vi "Problemas de Monitoreo.vi"() -> ()   [LabVIEW 2020]
uses:
  <vilib>/Instr/_visa.llb/VISA Configure Serial Port (Instr).vi
panel:
  out "Numeric":dbl
  in  "stop":bool
  out "string 3":string
  in  "string":string
  in  "Boolean 2":bool
  in  "Boolean":bool
  in  "VISA resource name":refnum<visa-resource-name>
  out "concatenated string":string
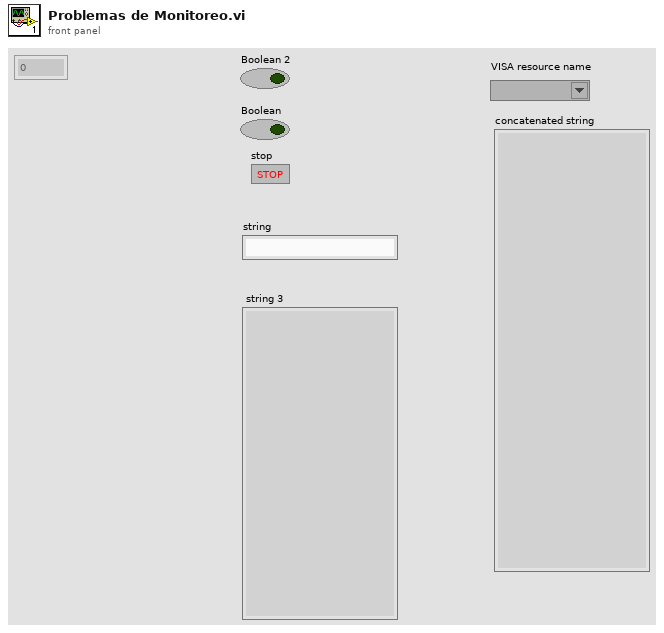
[diagram p1: front panel]
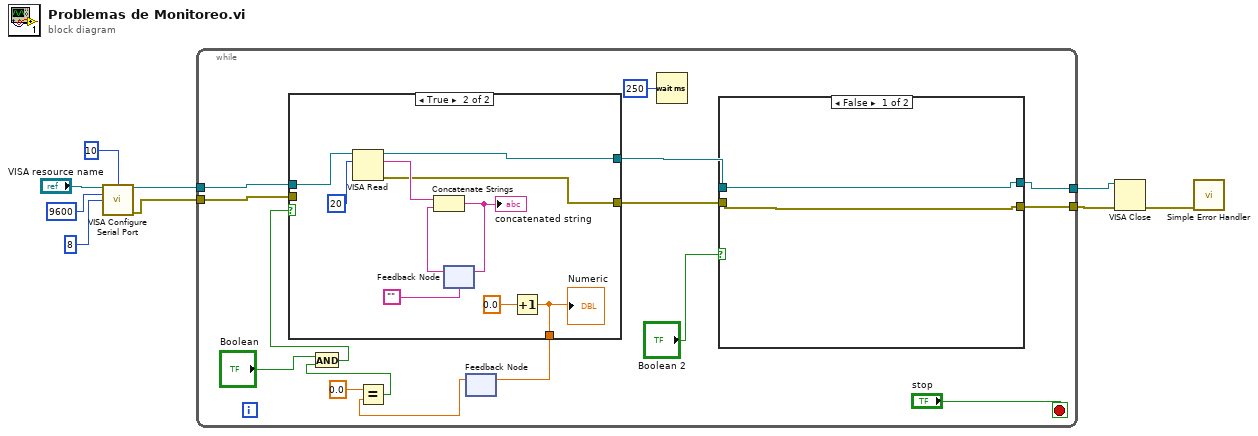
[diagram p0: block diagram]
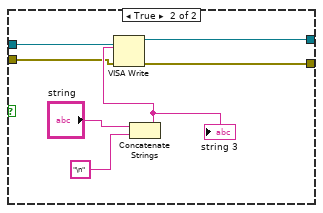
[diagram p2: hidden frame]
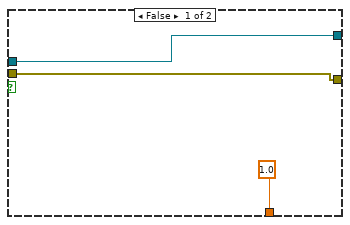
[diagram p3: hidden frame]
diagram:
  n1 = call-poly "VISA Configure Serial Port"("VISA resource name"="VISA resource name", "termination char\n(0xA = '\\n' = LF)"=u8 10 ("termination char\n(0xA = '\\n' = LF)"), "baud rate (9600)"=u32 9600, "data bits (8)"=u16 8) -> ("VISA resource name out"=w9:refnum<visa-resource-name>, "error out"=w3:errorcluster)  [unwired: 10 in]
  n2 = while {
    tunnel: w9 -> [w24]
    tunnel: [w22] -> w5
    tunnel: [w21] -> w4
    tunnel: w3 -> [w19]
    stop <- "stop" stop-if-true
    n3 = feedback #1() -> (w12:dbl)  [unwired: 1 in]
    n4 = Equal?(x=0.0, y=w12) -> (x = y?=w11:bool)
    n5 = And(x="Boolean", y=w11) -> (x .and. y?=w10:bool)
    n6 = case shown="True" w10 {
      tunnel: w24 -> [w36 w44]
      tunnel: [w36 w40] -> w20
      tunnel: [w35 w39] -> w18
      tunnel: w19 -> [w35 _]
      tunnel: [1.0 w37] -> w13
      frame False {
      }
      frame True {
        n7 = VISA Read(VISA resource name=w44, byte count=u32 20) -> (VISA resource name out=w40:refnum<visa-resource-name>, read buffer=w45:string, error out=w39:errorcluster)  [unwired: 1 in, 1 out]
        n8 = feedback #2("") -> (w43:string)
        n9 = Concatenate Strings(w45, w43) -> (w41:string)
        "concatenated string" <- w41
        n10 = feedback-in #2(w41) -> ()
        n11 = Increment(x=0.0) -> (x+1=w37:dbl)
        "Numeric" <- w37
      }
    }
    n12 = feedback-in #1(w13) -> ()
    n13 = Wait (ms)(milliseconds to wait=u32 250) -> ()  [unwired: 1 out]
    n14 = case shown="False" "Boolean 2" {
      tunnel: [w26 w30] -> w22
      tunnel: [w25 w29] -> w21
      tunnel: w20 -> [w26 w28]
      tunnel: w18 -> [w25 w27]
      frame False {
      }
      frame True {
        n15 = Concatenate Strings("string", "\n" ("string")) -> (w31:string)
        "string 3" <- w31
        n16 = VISA Write(VISA resource name=w28, write buffer=w31, error in (no error)=w27) -> (VISA resource name out=w30:refnum<visa-resource-name>, error out=w29:errorcluster)  [unwired: 1 out]
      }
    }
  }
  n17 = VISA Close(VISA resource name=w5, error in (no error)=w4) -> (error out=w1:errorcluster)
  n18 = call <vilib>:"Simple Error Handler.vi"("error in (no error)"=w1) -> ()  [unwired: 4 in, 5 out]
